vi "Tektronix TDS 3000 Series Transfer Current Waveform Example.vi"() -> ()   [LabVIEW 2010]
doc: "DESCRIPTION:\nThis example shows how to transfer the current waveform on an oscilloscope. Users can setup the acquired waveform using the instrument's front panel interface and then transfer that waveform to the computer using this example.\n\nINSTRUCTIONS:\n1. Pass a valid VISA session.\n2. Enter the desired channel.\n3. The acquired waveform will be displayed in the graph."
uses:
  <instrlib>/Tektronix TDS 3000 Series/Tektronix TDS 3000 Series.lvlib
panel:
  out "Waveform Graph":T1(graph)
  in  "Instrument Resource Name":refnum<visa-resource-name>="GPIB0::1::INSTR"
  in  "Serial Settings":T2={"Baud Rate (9600)"=9600, "Flow Control (RTS/CTS)"=2, "Data Bits (8)"=8} {"Flow Control (RTS/CTS)" items=["None"=0, "RTS/CTS"=2]; "Baud Rate (9600)" items=["1200"=1200, "2400"=2400, "4800"=4800, "9600"=9600, "19200"=19200, "38400"=38400]}
  # "© 2003-2006, National Instruments, Corporation.  All Rights Reserved."
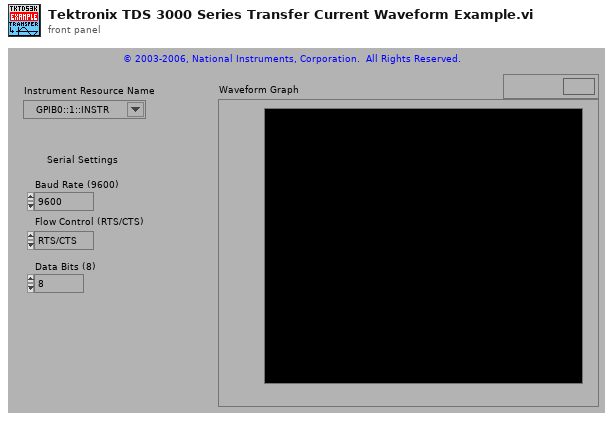
[diagram p1: front panel]
types:
  T1 = cluster{"Initial X":dbl, "X Increment":dbl, "Waveform Array":dbl[]}
  T2 = cluster{"Baud Rate (9600)":u32, "Flow Control (RTS/CTS)":u16, "Data Bits (8)":u16}
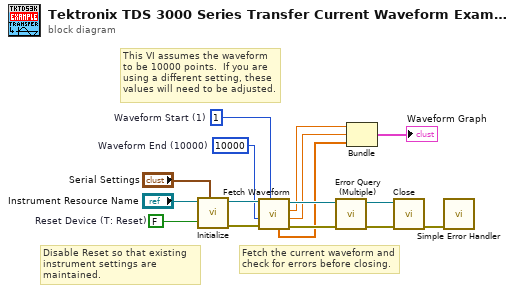
[diagram p0: block diagram]
diagram:
  w6 = 10000  # Waveform End (10000)
  w7 = 1  # Waveform Start (1)
  w8 = FALSE  # Reset Device (T: Reset)
  # "Fetch the current waveform and check for errors before closing."
  # "This VI assumes the waveform to be 10000 points.  If you are using a different setting, these values will need to be adjusted."
  # "Disable Reset so that existing instrument settings are maintained."
  n1 = call <instrlib>:"Initialize.vi"("Serial Settings"="Serial Settings", "Reset Device (T: Reset)"=w8, "VISA Resource Name"="Instrument Resource Name") -> ("error out"=w12:errorcluster, "VISA Resource Name Out"=w11:refnum<visa-resource-name>)  [unwired: 7 in]
  n2 = call <instrlib>:"Fetch Waveform.vi"("Waveform Start (1)"=w7, "error in (no error)"=w12, "Waveform End (10000)"=w6, "VISA Resource Name"=w11) -> ("error out"=w13:errorcluster, "X Increment"=w3:dbl, "Initial X"=w4:dbl, "VISA Resource Name Out"=w14:refnum<visa-resource-name>, "Waveform Array"=w2:dbl[])  [unwired: 2 in, 1 out]
  n3 = call <instrlib>:"Error Query (Multiple).vi"("error in (no error)"=w13, "VISA Resource Name"=w14) -> ("error out"=w15:errorcluster, "VISA Resource Name Out"=w16:refnum<visa-resource-name>)  [unwired: 6 in, 2 out]
  n4 = Bundle("Initial X"=w4, "X Increment"=w3, "Waveform Array"=w2) -> (→"Waveform Graph":T1)  [unwired: 1 in]
  n5 = call <instrlib>:"Close.vi"("error in (no error)"=w15, "VISA Resource Name"=w16) -> ("error out"=w5:errorcluster)  [unwired: 9 in]
  n6 = call <vilib>:"Simple Error Handler.vi"("error in (no error)"=w5) -> ()  [unwired: 4 in, 5 out]
